vi "Fatal.vi"(8 "Error In":errorcluster, 11 "Text":string) -> (0 "Error Out":errorcluster)   [LabVIEW 2015, in "Logger.lvlib"]
uses:
  Logger.lvlib
  Private/Action.ctl
  Controls/Message.ctl
  Controls/Tag.ctl
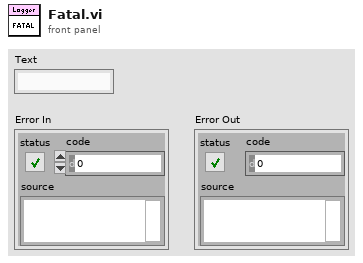
[diagram p1: front panel]
types:
  T1 = typedef "Logger.lvlib/Tag.ctl" = enum16{"Fatal", "Error", "Warn", "Info", "Debug", "Trace"}
  T2 = typedef "Logger.lvlib/Message.ctl" = cluster{"Time Stamp":timestamp, "Tag":T1, "Source":string, "Text":string}
  T3 = typedef "Logger.lvlib/Action.ctl" = enum16{"Initialize", "Register", "Log", "Unregister", "Set Level", "Shutdown"}
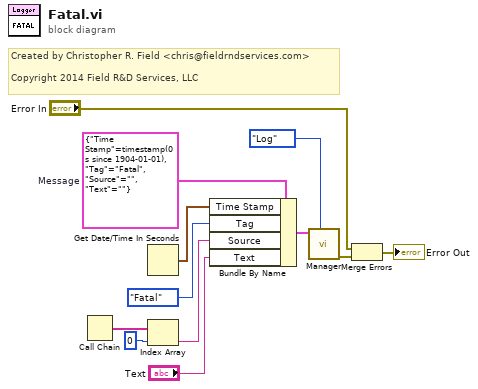
[diagram p0: block diagram]
diagram:
  w8 = T2 {"Time Stamp"=timestamp(0 s since 1904-01-01), "Tag"=enum."Fatal", "Source"="", "Text"=""}  # Message
  # "Created by Christopher R. Field <chris@fieldrndservices.com>\n\nCopyright 2014 Field R&D Services, LLC"
  n1 = Call Chain() -> (call chain=w10:string[])
  n2 = Get Date/Time In Seconds() -> (seconds since 1Jan1904=w7:timestamp)
  n3 = Index Array(array=w10, index=0) -> (element=w5:string)
  n4 = Bundle By Name(cluster=w8, "Time Stamp"=w7, "Tag"=Tag."Fatal" ("Level"), "Source"=w5, "Text"="Text") -> (w4:T2)
  n5 = call "Manager.vi"("Action"=Action."Log", "Value In"=w4) -> ("Error Out"=w3:errorcluster)  [unwired: 9 in]
  n6 = Merge Errors("Error In", w3) -> (→"Error Out":errorcluster)
